vi "Write Processes.vi"(8 "error in (no error)":errorcluster, 10 "Processes":refnum<vi>[](array[refnum]), 11 "Maui Manager in":refnum<class "Maui Manager.lvclass">) -> (0 "error out":errorcluster, 3 "Maui Manager out":refnum<class "Maui Manager.lvclass">)   [LabVIEW 2019, in "Maui Manager.lvclass"]
uses:
  Maui Manager.lvclass
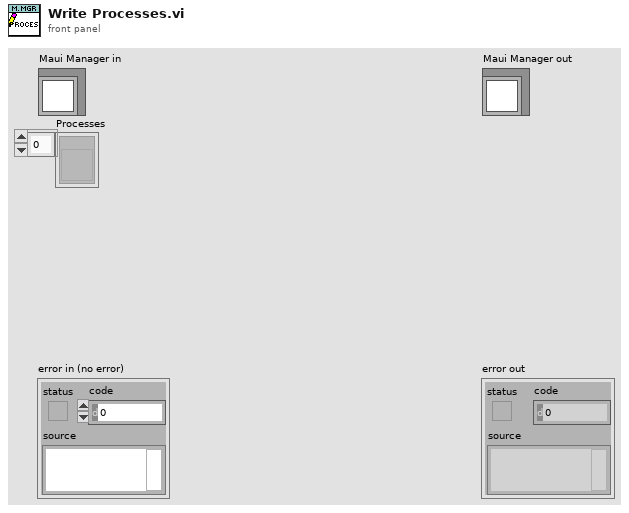
[diagram p1: front panel]
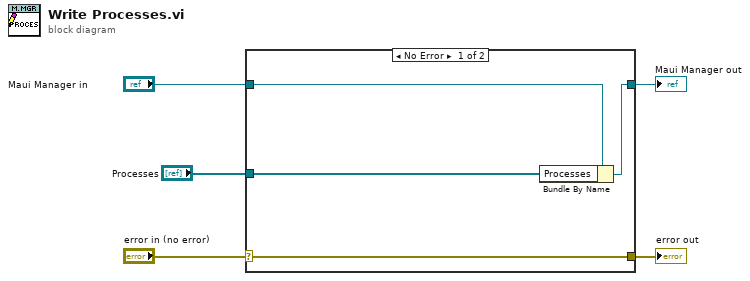
[diagram p0: block diagram]
diagram:
  n1 = case shown="No Error" "error in (no error)" {
    selector: "error in (no error)" -> [w9 w10]
    tunnel: [w9 w10] -> w4
    tunnel: [w7 w11] -> w2
    tunnel: "Maui Manager in" -> [w8 w11]
    tunnel: "Processes" -> [w6 _]
    frame No Error {
      n2 = Bundle By Name(cluster=w8, "Processes"=w6) -> (w7:refnum<class "Maui Manager.lvclass">)
    }
    frame Error {
    }
  }
  "error out" <- w4
  "Maui Manager out" <- w2
